vi "Msgbox - Save Status.vi"(6 "Simulate Fail":bool, 8 "error in (no error)":errorcluster, 9 "{Save ....} Failed":string="{Save User} Failed.", 10 "Control Value":string, 11 "{Save .....} [.....] =":string="{Save User} [UserId] = ") -> (0 "error out":errorcluster)   [LabVIEW 2013]
uses:
  Controls/Message Code - Enum.ctl
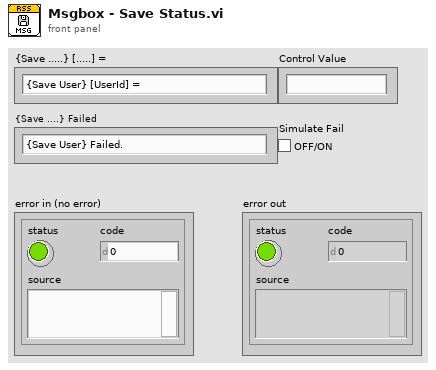
[diagram p1: front panel]
types:
  T1 = typedef "Message Code - Enum.ctl" = enum16{"<APP><I 100>", "<APP><E 101>", "<APP><I 110>", "<APP><W 111>", "<APP><I 112>", "<APP><W 113>", "<APP><I 114>", "<APP><I 115>", "<APP><I 116>", "<APP><W 117>", "<APP><I 120>", "<APP><W 121>", "<APP><E 122>", "<APP><W 130>", "<APP><W 131>", "<APP><W 132>", "<APP><W 133>", "<APP><W 134>", "<DB><I 150>", "<DB><I 151>", "<DB><W 152>", "<APP><I 200>", "<APP><I 201>", "<APP><W 202>", "<APP><E 203>", "<DB><I 300>", "<DB><I 301>", "<DB><W 302>", "<DB><I 305>", "<DB><I 306>", "<DB><W 307>", "<DB><W 310>", "<cRIO><I 400>", "<cRIO><W 401>", "<cRIO><I 402>", "<cRIO><W 403>", "<ET><I 500>", "<ET><W 501>", "<ET><I 600>", "<ET><W 601>", "<ET><E 602>", "<ET><I 610>", "<ET><W 611>", "<ET><E 612>"}
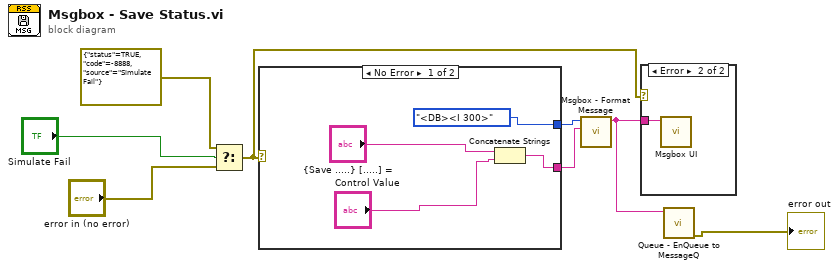
[diagram p0: block diagram]
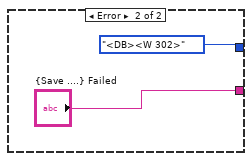
[diagram p2: hidden frame]
diagram:
  n1 = Select(t=errorcluster {"status"=TRUE, "code"=-8888, "source"="Simulate Fail"}, s="Simulate Fail", f="error in (no error)") -> (s? t:f=w7:errorcluster)
  n2 = case shown="No Error" w7 {
    tunnel: [Message_Code_-_Enum."<DB><I 300>" ("Message Code\n2014-10-01") Message_Code_-_Enum."<DB><W 302>" ("Message Code\n2014-10-01")] -> w5
    tunnel: [w10 "{Save ....} Failed"] -> w6
    frame No Error {
      n3 = Concatenate Strings("{Save .....} [.....] =", "Control Value") -> (w10:string)
    }
    frame Error {
    }
  }
  n4 = call "Msgbox - Format Message.vi"("Message"=w6, "Message Code\n2014-10-01"=w5) -> ("Message"=w4:string)  [unwired: 8 in, 1 out]
  n5 = case shown="Error" w7 {
    tunnel: w4 -> [_ w15]
    frame No Error {
    }
    frame Error {
      n6 = call "Msgbox UI.vi"("[MessageType]"=w15) -> ()  [unwired: 8 in, 3 out]
    }
  }
  n7 = call "Queue - EnQueue to MessageQ.vi"("Message"=w4) -> ("Error Out"=→"error out":errorcluster)  [unwired: 10 in]
